vi "test_FgenInstrument_CallInitializeMeasurementLinkSessionWithCreateBehavior_RemoteSessionCreated.vi"(8 "error in":errorcluster) -> (0 "error out":errorcluster, 2 "result":string, 3 "pass":bool)   [LabVIEW 2020, in "MeasurementServerTests.lvlib"]
uses:
  MeasurementServerTests.lvlib
  Runtime/Sessions/niFGEN Sessions/Session Factory/Session Factory.lvclass
  Runtime/Sessions/Instrument Sessions/ISession Factory/Initialize and Close Session Behavior.ctl
  Runtime/Sessions/Instrument Sessions/ISession Factory/ISession Factory.lvclass
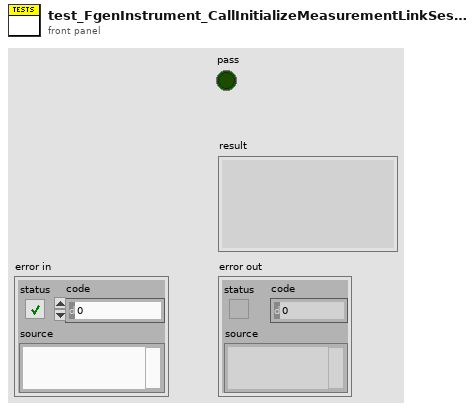
[diagram p1: front panel]
types:
  T1 = typedef "Instrument Sessions.lvlib/ISession Factory.lvclass/Remote Connection Options.ctl" = cluster{"session name":string, "address":string, "port":u32}
  T2 = typedef "Instrument Sessions.lvlib/ISession Factory.lvclass/Initialize and Close Session Behavior.ctl" = enum16{"Initialize and Close", "Attach and Detach", "Initialize and Detach", "Attach and Close"}
  T3 = typedef "Instrument Sessions.lvlib/ISession Factory.lvclass/Session Initialization Parameters.ctl" = cluster{"resource name":string, "session name":string}
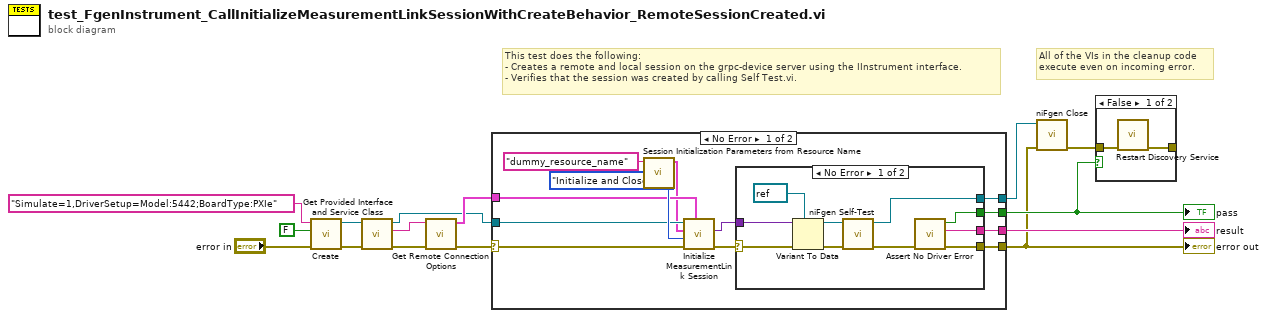
[diagram p0: block diagram]
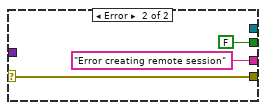
[diagram p2: hidden frame]
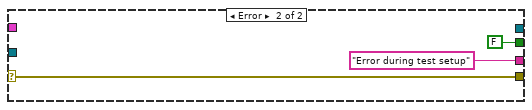
[diagram p3: hidden frame]
diagram:
  # "All of the VIs in the cleanup code\nexecute even on incoming error."
  # "This test does the following:\n- Creates a remote and local session on the grpc-device server using the IInstrument interface.\n- Verifies that the session was created by calling Self Test.vi."
  n1 = call "Create.vi"("error in"="error in", "reset"=FALSE, "option string"="Simulate=1,DriverSetup=Model:5442;BoardType:PXIe") -> ("error out"=w5:errorcluster, "session factory out"=w4:refnum<class "Session Factory.lvclass">)  [unwired: 7 in]
  n2 = call-dynamic "Get Provided Interface and Service Class.vi"("error in"=w5, "session factory in"=w4) -> ("error out"=w13:errorcluster, "provided interface"=w14:string, "session factory out"=w10:refnum<class "Session Factory.lvclass">)  [unwired: 6 in, 1 out]
  n3 = call "Get Remote Connection Options.vi"("error in"=w13, "provided interface"=w14) -> ("error out"=w12:errorcluster, "remote connection options"=w11:T1)  [unwired: 8 in]
  n4 = case shown="No Error" w12 {
    selector: w12 -> [w20 w41]
    tunnel: [w26 w41] -> w7
    tunnel: [w27 FALSE] -> w8
    tunnel: [w25 "Error during test setup" ("f")] -> w15
    tunnel: w11 -> [w19 _]
    tunnel: w10 -> [w18 _]
    tunnel: [w17 _] -> w2
    frame No Error {
      n5 = call "Session Initialization Parameters from Resource Name.vi"("resource name"="dummy_resource_name") -> ("session initialization parameters"=w16:T3)  [unwired: 10 in]
      n6 = call-dynamic "Initialize MeasurementLink Session.vi"("remote connection options"=w19, "error in"=w20, "initialize and close session behavior"=Initialize_and_Close_Session_Behavior."Initialize and Close", "session initialization parameters"=w16, "session factory in"=w18) -> ("error out"=w23:errorcluster, "session out"=w24:variant)  [unwired: 4 in, 1 out]
      n7 = case shown="No Error" w23 {
        selector: w23 -> [w36 w39]
        tunnel: [w28 FALSE] -> w27
        tunnel: [w30 w39] -> w26
        tunnel: [w29 "Error creating remote session"] -> w25
        tunnel: w24 -> [w37 _]
        tunnel: [w32 _] -> w17
        frame No Error {
          n8 = Variant To Data(error in=w36, type=refnum<k15> refnum ("Instrument Handle Out"), Variant=w37) -> (data=w34:refnum<k15>, error out=w35:errorcluster)
          n9 = call <instrlib>:"niFgen Self-Test.vi"("error in (no error)"=w35, "Instrument Handle"=w34) -> ("error out"=w31:errorcluster, "Instrument Handle Out"=w32:refnum<k15>)  [unwired: 6 in, 2 out]
          n10 = call "Assert No Driver Error.vi"("error in"=w31) -> ("error out"=w30:errorcluster, "result"=w29:string, "pass?"=w28:bool)  [unwired: 8 in]
        }
        frame Error {
        }
      }
    }
    frame Error {
    }
  }
  "error out" <- w7
  "pass" <- w8
  "result" <- w15
  n11 = call <instrlib>:"niFgen Close.vi"("error in (no error)"=w7, "Instrument Handle"=w2) -> ("error out"=w9:errorcluster)  [unwired: 9 in]
  n12 = case shown="False" w8 {
    tunnel: w9 -> [w45 _]
    tunnel: [w44 _] -> _
    frame False {
      n13 = call "Restart Discovery Service.vi"("error in"=w45) -> ("error out"=w44:errorcluster)  [unwired: 10 in]
    }
    frame True {
    }
  }
